vi "Convert_to_number2.vi"(2 "Array - String":string[](array[string]), 4 "string":string) -> (0 "Number":dbl format="%.2f", 1 "offset past number":i32)   [LabVIEW 2022 SP3]
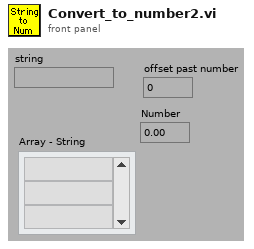
[diagram p1: front panel]
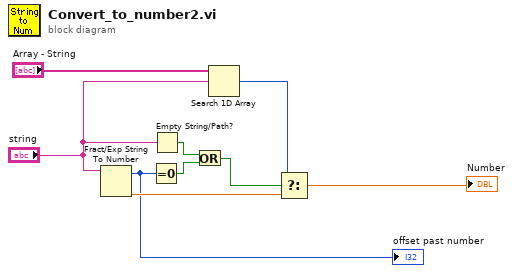
[diagram p0: block diagram]
diagram:
  n1 = Fract/Exp String To Number(string="string") -> (offset past number=w7:i32, number=w9:dbl)  [unwired: 3 out]
  "offset past number" <- w7
  n2 = Equal To 0?(x=w7) -> (x = 0?=w6:bool)
  n3 = Empty String/Path?(string/path="string") -> (empty?=w5:bool)
  n4 = Or(x=w5, y=w6) -> (x .or. y?=w4:bool)
  n5 = Search 1D Array(1D array="Array - String", element="string") -> (index of element=w1:i32)  [unwired: 1 in]
  n6 = Select(t=w1, s=w4, f=w9) -> (s? t:f=→"Number":dbl)
